vi "Init Root Actors.vi"(6 "Core Actors":refnum<class "Actor.lvclass">[](array[class]), 9 "Mid Actors":refnum<class "Actor.lvclass">[](array[class]), 10 "Edge Actors":refnum<class "Actor.lvclass">[](array[class])) -> (2 "Root Actors":refnum<class "Root Actors.lvclass">)   [LabVIEW 2020, in "jettl.lvlib" / "Base Root Actors.lvlib"]
uses:
  Base Root Actors.lvlib
  Root Actors/Root Actors.lvclass
  Actor/Actor.lvclass
  Base Root Actors/Base Root Actors.lvclass
  C:/git/jettl/src/jettl/jettl/Root Actors/Root Actors.lvclass
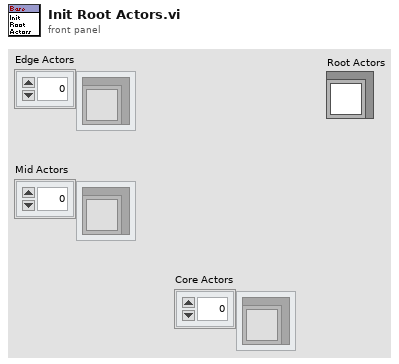
[diagram p1: front panel]
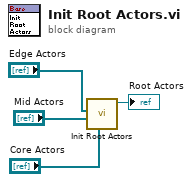
[diagram p0: block diagram]
diagram:
  n1 = call "Init Root Actors.vi"("Core Actors"="Core Actors", "Mid Actors"="Mid Actors", "Edge Actors"="Edge Actors") -> ("Base Root Actors out"=→"Root Actors":refnum<class "Base Root Actors.lvclass">)  [unwired: 8 in]
